vi "MagBoard_n128_Init_Board.vi"(8 "error in (no error)":errorcluster, 10 "Serial Settings":T1={"baud rate"=115200, "data bits"=8, "parity"=enum."None", "stop bits"=10, "flow control"=0} {"flow control" items=["None"=0, "XON/XOFF"=1, "RTS/CTS"=2, "DTR/DSR"=4]; "stop bits" items=["1.0"=10, "1.5"=15, "2.0"=20]; "data bits" min=5 max=8 step=1; "baud rate" items=["75"=75, "110"=110, "134"=134, "150"=150, "300"=300, "600"=600, "1200"=1200, "1800"=1800, "2400"=2400, "4800"=4800, "7200"=7200, "9600"=9600, "14400"=14400, "19200"=19200, "28800"=28800, "38400"=38400, "56000"=56000, "57600"=57600, "115200"=115200, "128000"=128000, "230400"=230400]}, 11 "VISA resource name":refnum<visa-resource-name>="COM16") -> (0 "error out":errorcluster)   [LabVIEW 2018]
panel:
  in  "Tab Control":enum32{"Display", "Configuration"}(tab)
  out "Connected":bool
  out "Initialised":bool
  out "Init string":string
  # "scapes: Connection"
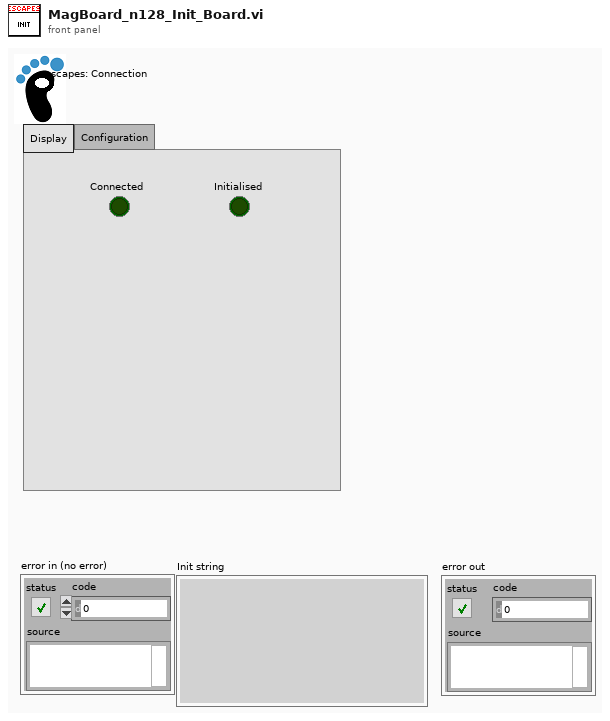
[diagram p1: front panel]
types:
  T1 = cluster{"baud rate":u32, "data bits":u16, "parity":enum16{"None", "Odd", "Even", "Mark", "Space"}, "stop bits":u16, "flow control":u16}
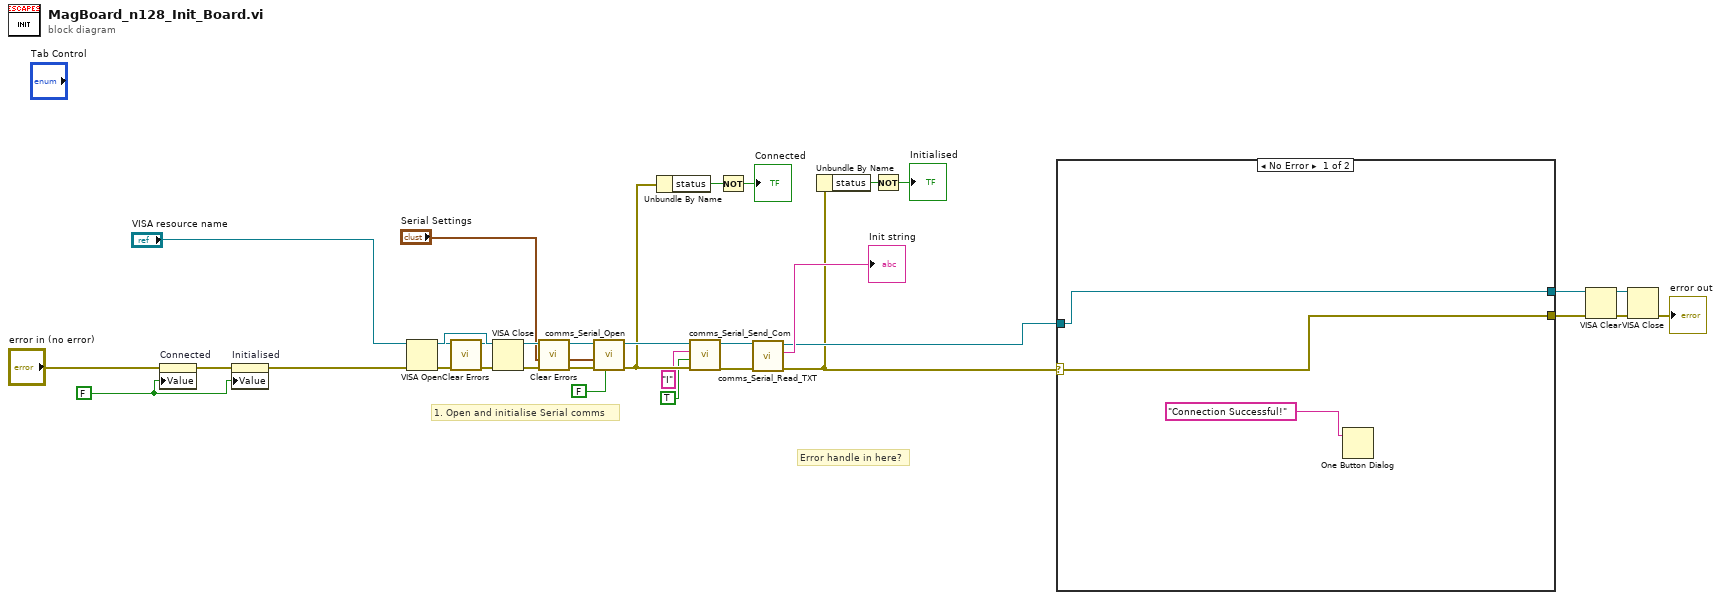
[diagram p0: block diagram]
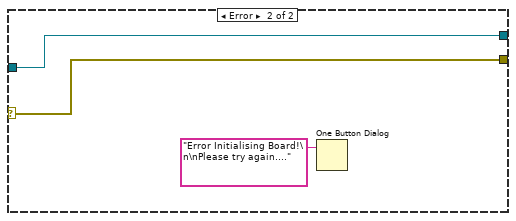
[diagram p2: hidden frame]
diagram:
  w16 = FALSE ("Send Init Comm?")
  # "Error handle in here?"
  # "1. Open and initialise Serial comms"
  n1 = property on="Connected" class="Bool (strict)"(error in="error in (no error)", "Value"=w16) -> (error out=w17:errorcluster)  [unwired: 1 in, 1 out]
  n2 = property on="Initialised" class="Bool (strict)"(error in=w17, "Value"=w16) -> (error out=w2:errorcluster)  [unwired: 1 in, 1 out]
  n3 = VISA Open(error in (no error)=w2, VISA resource name="VISA resource name") -> (VISA resource name=w15:refnum<visa-resource-name>, error out=w14:errorcluster)  [unwired: 3 in]
  n4 = call <vilib>:"Clear Errors.vi"("error in (no error)"=w14) -> ("error out"=w13:errorcluster)  [unwired: 5 in, 1 out]
  n5 = VISA Close(VISA resource name=w15, error in (no error)=w13) -> (error out=w12:errorcluster)
  n6 = call <vilib>:"Clear Errors.vi"("error in (no error)"=w12) -> ("error out"=w11:errorcluster)  [unwired: 5 in, 1 out]
  n7 = call "comms_Serial_Open.vi"("Send Init Comm?"=FALSE, "error in (no error)"=w11, "Serial Settings in"="Serial Settings", "VISA Refnum in"="VISA resource name") -> ("error out"=w22:errorcluster, "VISA Refnum out"=w24:refnum<visa-resource-name>)  [unwired: 5 in, 1 out]
  n8 = Unbundle By Name(w22) -> ("status"=w21:bool)
  n9 = call "comms_Serial_Send_Com.vi"("Buffer Clear?"=TRUE, "Command"="I", "VISA resource in"=w24) -> ("VISA resource Out"=w3:refnum<visa-resource-name>)  [unwired: 6 in, 2 out]
  n10 = Not(x=w21) -> (.not. x?=→"Connected":bool)
  n11 = call "comms_Serial_Read_TXT.vi"("error in"=w22, "VISA resource in"=w3) -> ("error out"=w6:errorcluster, "Data Out"=→"Init string":string, "VISA resource Out"=w7:refnum<visa-resource-name>)  [unwired: 6 in, 1 out]
  n12 = Unbundle By Name(w6) -> ("status"=w20:bool)
  n13 = Not(x=w20) -> (.not. x?=→"Initialised":bool)
  n14 = case shown="No Error" w6 {
    selector: w6 -> [w31 w34]
    tunnel: [w32 w35] -> w26
    tunnel: [w31 w34] -> w25
    tunnel: w7 -> [w32 w35]
    frame No Error {
      n15 = One Button Dialog(message="Connection Successful!") -> ()  [unwired: 1 in, 1 out]
    }
    frame Error {
      n16 = One Button Dialog(message="Error Initialising Board!\n\nPlease try again....") -> ()  [unwired: 1 in, 1 out]
    }
  }
  n17 = VISA Clear(VISA resource name=w26, error in (no error)=w25) -> (VISA resource name out=w28:refnum<visa-resource-name>, error out=w27:errorcluster)
  n18 = VISA Close(VISA resource name=w28, error in (no error)=w27) -> (error out=→"error out":errorcluster)
